vi "load_conditions.vi"(0 "VI's Path":path, 2 "Load Type":string(combo), 7 "Config In":T1, 11 "error in":errorcluster) -> (8 "Config Out":T1, 15 "error out":errorcluster)   [LabVIEW 2023]
uses:
  <vilib>/Utility/config.llb/Read Key (Double).vi
  <vilib>/Utility/config.llb/Read Key (Boolean).vi
  <vilib>/Utility/config.llb/NI_LVConfig.lvlib
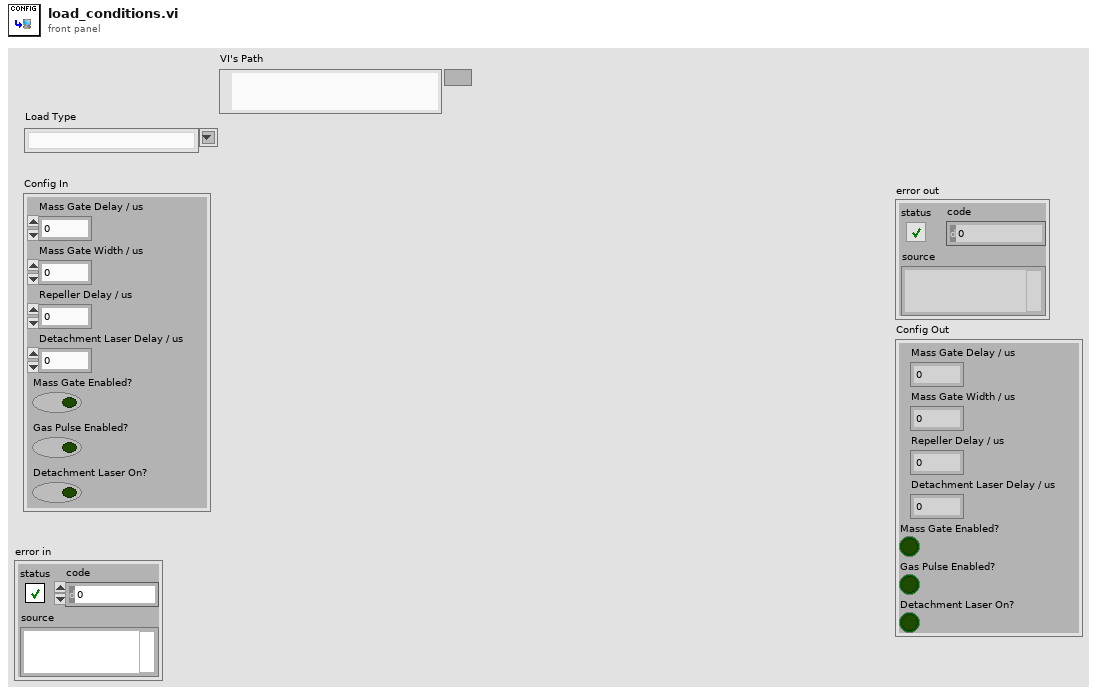
[diagram p1: front panel]
types:
  T1 = cluster{"Mass Gate Delay / us":dbl, "Mass Gate Width / us":dbl, "Repeller Delay / us":dbl, "Detachment Laser Delay / us":dbl, "Mass Gate Enabled?":bool, "Gas Pulse Enabled?":bool, "Detachment Laser On?":bool}
  T2 = typedef "NI_LVConfig.lvlib/Config Data RefNum.ctl" = refnum<k1>
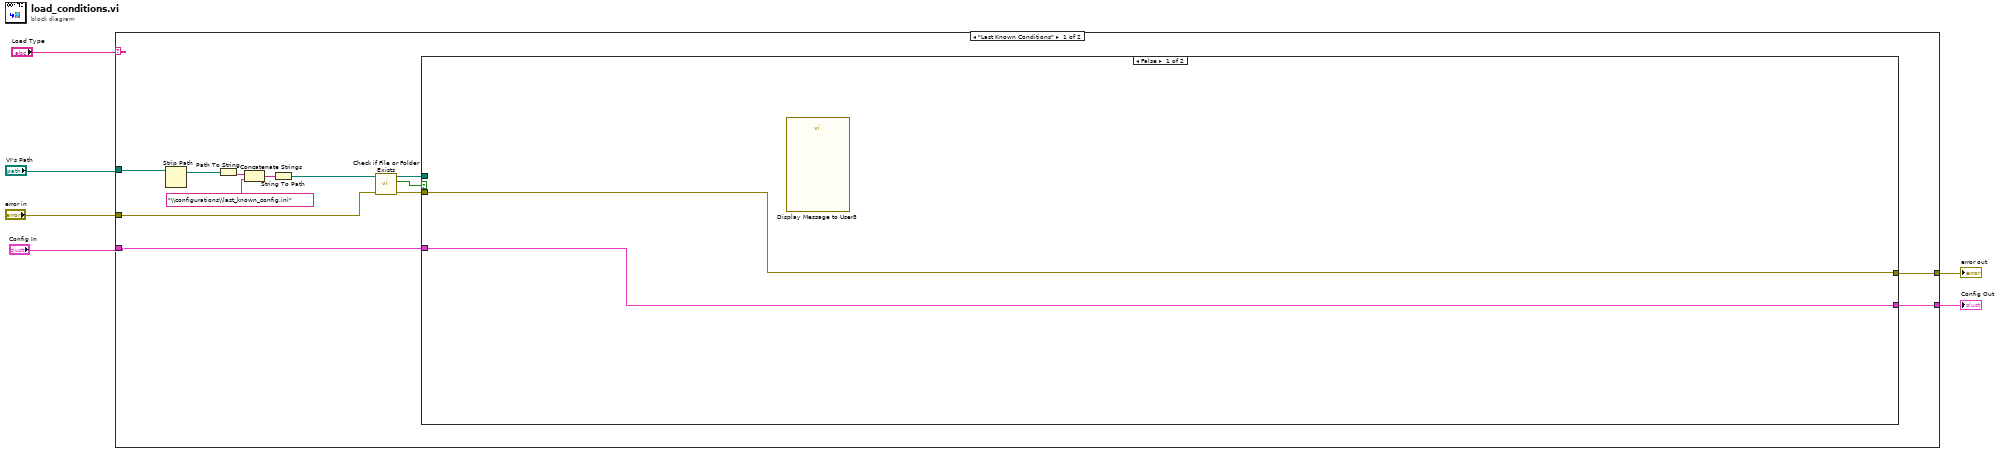
[diagram p0: block diagram]
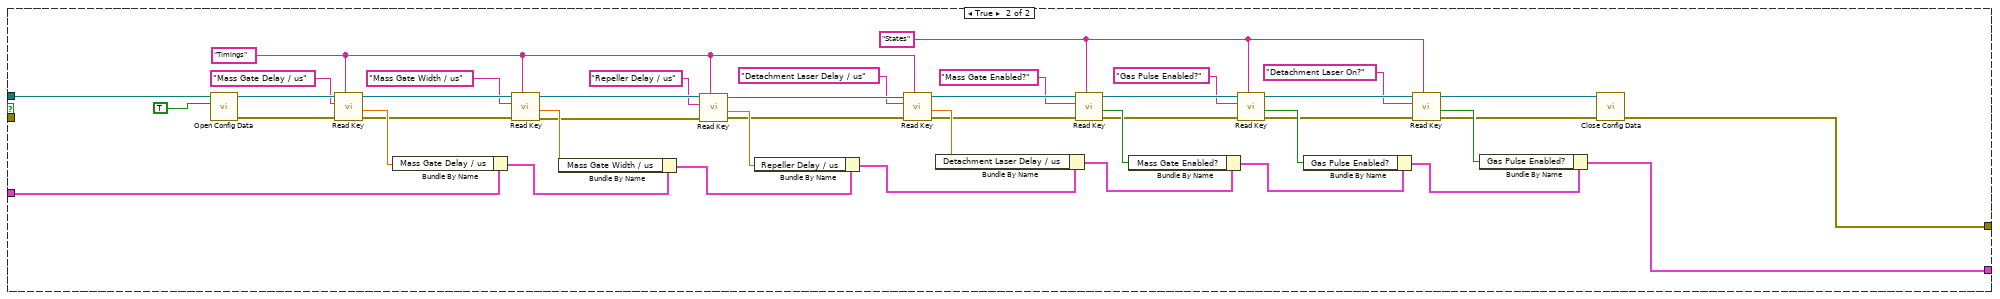
[diagram p2: hidden frame]
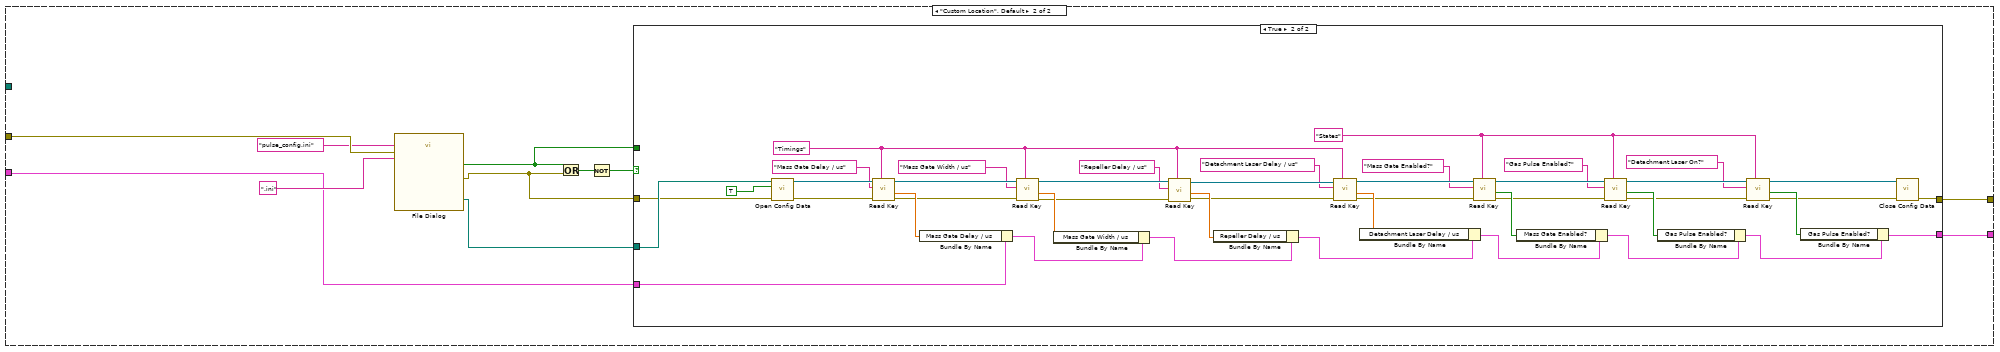
[diagram p3: hidden frame]
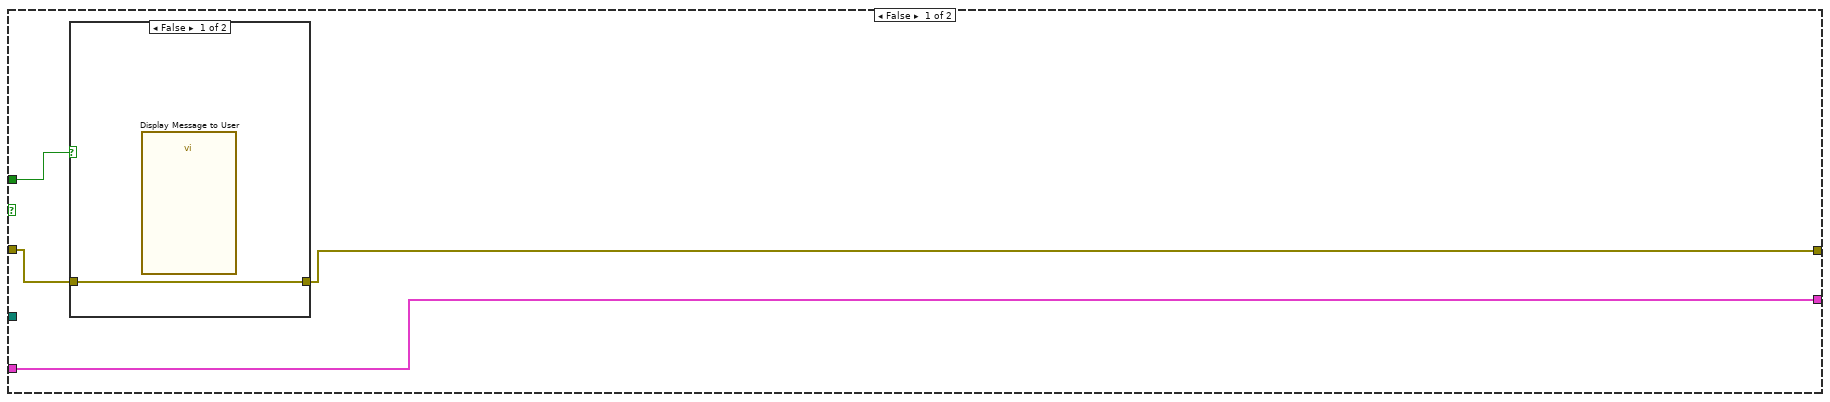
[diagram p4: hidden frame]
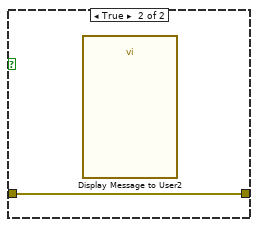
[diagram p5: hidden frame]
diagram:
  n1 = case shown="\"Last Known Conditions\"" "Load Type" {
    tunnel: "error in" -> [w13 w70]
    tunnel: [w7 w67] -> w5
    tunnel: "Config In" -> [w9 w66]
    tunnel: [w8 w65] -> w3
    tunnel: "VI's Path" -> [w19 _]
    frame "Last Known Conditions" {
      n2 = Strip Path(path=w19) -> (stripped path=w15:path)  [unwired: 1 out]
      n3 = Path To String(path=w15) -> (string=w18:string)
      n4 = Concatenate Strings(w18, "\\configurations\\last_known_config.ini" ("string")) -> (w16:string)
      n5 = String To Path(string=w16) -> (path=w14:path)
      n6 = call <vilib>:"Check if File or Folder Exists.vi"("error in (no error)"=w13, "path"=w14) -> ("error out"=w10:errorcluster, "file or folder exists?"=w12:bool, "dup path"=w11:path)  [unwired: 7 in]
      n7 = case shown="False" w12 {
        tunnel: w11 -> [_ w25]
        tunnel: w10 -> [w20 _]
        tunnel: w9 -> [w21 w24]
        tunnel: [w21 w23] -> w8
        tunnel: [w20 w22] -> w7
        frame False {
          n8 = call "Display Message to User3"() -> ()  [unwired: 10 in, 2 out]
        }
        frame True {
          w32 = "States" ("section")
          w48 = "Timings" ("section")
          n9 = call <vilib>:"Open Config Data.vi"("create file if necessary (T)"=TRUE, "configuration file path"=w25) -> ("error out"=w62:errorcluster, "refnum"=w63:T2)  [unwired: 7 in, 1 out]
          n10 = call-poly <vilib>:"Read Key.vi"("section"=w48, "error in (no error)"=w62, "key"="Mass Gate Delay / us", "refnum"=w63) -> ("error out"=w58:errorcluster, "value"=w60:dbl, "refnum out"=w59:T2)  [unwired: 4 in, 1 out]
          n11 = Bundle By Name(cluster=w24, "Mass Gate Delay / us"=w60) -> (w51:T1)
          n12 = call-poly <vilib>:"Read Key.vi"("section"=w48, "error in (no error)"=w58, "key"="Mass Gate Width / us", "refnum"=w59) -> ("error out"=w54:errorcluster, "value"=w56:dbl, "refnum out"=w55:T2)  [unwired: 4 in, 1 out]
          n13 = Bundle By Name(cluster=w51, "Mass Gate Width / us"=w56) -> (w42:T1)
          n14 = call-poly <vilib>:"Read Key.vi"("section"=w48, "error in (no error)"=w54, "key"="Repeller Delay / us", "refnum"=w55) -> ("error out"=w49:errorcluster, "value"=w52:dbl, "refnum out"=w50:T2)  [unwired: 4 in, 1 out]
          n15 = Bundle By Name(cluster=w42, "Repeller Delay / us"=w52) -> (w41:T1)
          n16 = call-poly <vilib>:"Read Key.vi"("section"=w48, "error in (no error)"=w49, "key"="Detachment Laser Delay / us", "refnum"=w50) -> ("error out"=w40:errorcluster, "value"=w46:dbl, "refnum out"=w45:T2)  [unwired: 4 in, 1 out]
          n17 = Bundle By Name(cluster=w41, "Detachment Laser Delay / us"=w46) -> (w36:T1)
          n18 = call-poly <vilib>:"Read Key.vi"("section"=w32, "error in (no error)"=w40, "key"="Mass Gate Enabled?", "refnum"=w45) -> ("error out"=w38:errorcluster, "value"=w43:bool, "refnum out"=w39:T2)  [unwired: 4 in, 1 out]
          n19 = Bundle By Name(cluster=w36, "Mass Gate Enabled?"=w43) -> (w30:T1)
          n20 = call-poly <vilib>:"Read Key.vi"("section"=w32, "error in (no error)"=w38, "key"="Gas Pulse Enabled?", "refnum"=w39) -> ("error out"=w33:errorcluster, "value"=w35:bool, "refnum out"=w34:T2)  [unwired: 4 in, 1 out]
          n21 = Bundle By Name(cluster=w30, "Gas Pulse Enabled?"=w35) -> (w29:T1)
          n22 = call-poly <vilib>:"Read Key.vi"("section"=w32, "error in (no error)"=w33, "key"="Detachment Laser On?", "refnum"=w34) -> ("error out"=w26:errorcluster, "value"=w28:bool, "refnum out"=w27:T2)  [unwired: 4 in, 1 out]
          n23 = Bundle By Name(cluster=w29, "Gas Pulse Enabled?"=w28) -> (w23:T1)
          n24 = call <vilib>:"Close Config Data.vi"("error in (no error)"=w26, "refnum"=w27) -> ("error out"=w22:errorcluster)  [unwired: 8 in, 1 out]
        }
      }
    }
    frame "Custom Location", Default {
      n25 = call "File Dialog"("default name"="pulse_config.ini", "error in"=w70, "pattern (all files)"=".ini") -> ("selected path"=w71:path, "cancelled"=w72:bool, "error out"=w73:errorcluster)  [unwired: 9 in, 1 out]
      n26 = Or(x=w72, y=w73) -> (x .or. y?=w75:bool)
      n27 = Not(x=w75) -> (.not. x?=w74:bool)
      n28 = case shown="True" w74 {
        tunnel: w73 -> [w78 w123]
        tunnel: w72 -> [w79 _]
        tunnel: w71 -> [_ w124]
        tunnel: [w77 w82] -> w67
        tunnel: w66 -> [w76 w88]
        tunnel: [w76 w83] -> w65
        frame False {
          n29 = case shown="False" w79 {
            tunnel: [w80 w81] -> w77
            tunnel: w78 -> [w80 w81]
            frame False {
              n30 = call "Display Message to User"() -> ()  [unwired: 10 in, 2 out]
            }
            frame True {
              n31 = call "Display Message to User2"() -> ()  [unwired: 10 in, 2 out]
            }
          }
        }
        frame True {
          w91 = "States" ("section")
          w107 = "Timings" ("section")
          n32 = call <vilib>:"Open Config Data.vi"("error in (no error)"=w123, "create file if necessary (T)"=TRUE, "configuration file path"=w124) -> ("error out"=w121:errorcluster, "refnum"=w122:T2)  [unwired: 6 in, 1 out]
          n33 = call-poly <vilib>:"Read Key.vi"("section"=w107, "error in (no error)"=w121, "key"="Mass Gate Delay / us", "refnum"=w122) -> ("error out"=w117:errorcluster, "value"=w119:dbl, "refnum out"=w118:T2)  [unwired: 4 in, 1 out]
          n34 = Bundle By Name(cluster=w88, "Mass Gate Delay / us"=w119) -> (w110:T1)
          n35 = call-poly <vilib>:"Read Key.vi"("section"=w107, "error in (no error)"=w117, "key"="Mass Gate Width / us", "refnum"=w118) -> ("error out"=w113:errorcluster, "value"=w115:dbl, "refnum out"=w114:T2)  [unwired: 4 in, 1 out]
          n36 = Bundle By Name(cluster=w110, "Mass Gate Width / us"=w115) -> (w101:T1)
          n37 = call-poly <vilib>:"Read Key.vi"("section"=w107, "error in (no error)"=w113, "key"="Repeller Delay / us", "refnum"=w114) -> ("error out"=w108:errorcluster, "value"=w111:dbl, "refnum out"=w109:T2)  [unwired: 4 in, 1 out]
          n38 = Bundle By Name(cluster=w101, "Repeller Delay / us"=w111) -> (w100:T1)
          n39 = call-poly <vilib>:"Read Key.vi"("section"=w107, "error in (no error)"=w108, "key"="Detachment Laser Delay / us", "refnum"=w109) -> ("error out"=w99:errorcluster, "value"=w105:dbl, "refnum out"=w104:T2)  [unwired: 4 in, 1 out]
          n40 = Bundle By Name(cluster=w100, "Detachment Laser Delay / us"=w105) -> (w95:T1)
          n41 = call-poly <vilib>:"Read Key.vi"("section"=w91, "error in (no error)"=w99, "key"="Mass Gate Enabled?", "refnum"=w104) -> ("error out"=w97:errorcluster, "value"=w102:bool, "refnum out"=w98:T2)  [unwired: 4 in, 1 out]
          n42 = Bundle By Name(cluster=w95, "Mass Gate Enabled?"=w102) -> (w89:T1)
          n43 = call-poly <vilib>:"Read Key.vi"("section"=w91, "error in (no error)"=w97, "key"="Gas Pulse Enabled?", "refnum"=w98) -> ("error out"=w92:errorcluster, "value"=w94:bool, "refnum out"=w93:T2)  [unwired: 4 in, 1 out]
          n44 = Bundle By Name(cluster=w89, "Gas Pulse Enabled?"=w94) -> (w87:T1)
          n45 = call-poly <vilib>:"Read Key.vi"("section"=w91, "error in (no error)"=w92, "key"="Detachment Laser On?", "refnum"=w93) -> ("error out"=w84:errorcluster, "value"=w86:bool, "refnum out"=w85:T2)  [unwired: 4 in, 1 out]
          n46 = Bundle By Name(cluster=w87, "Gas Pulse Enabled?"=w86) -> (w83:T1)
          n47 = call <vilib>:"Close Config Data.vi"("error in (no error)"=w84, "refnum"=w85) -> ("error out"=w82:errorcluster)  [unwired: 8 in, 1 out]
        }
      }
    }
  }
  "error out" <- w5
  "Config Out" <- w3
